vi "CreateShearRampStepVisualizationGraph.vi"(8 "Step Duration":dbl, 9 "Final Value":dbl, 10 "Initial Value":dbl, 11 "Number of Points":i32) -> (2 "Shear Step Array":dbl[][](array[numeric]), 3 "XY Graph":cluster{dbl[], "Ramp Pattern":dbl[]}(graph))   [LabVIEW 2021]
uses:
  <vilib>/Analysis/1siggen.llb/Ramp Pattern by Samples.vi
  <vilib>/Analysis/NI_AALBase.lvlib
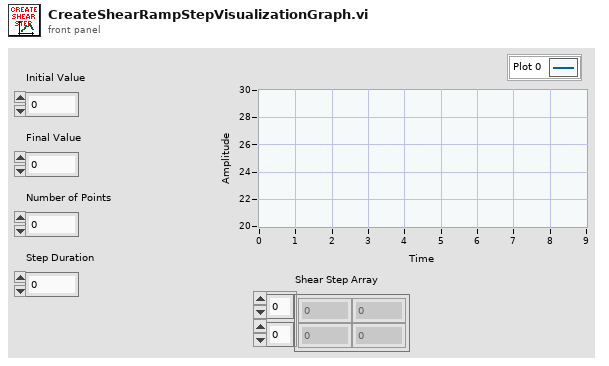
[diagram p1: front panel]
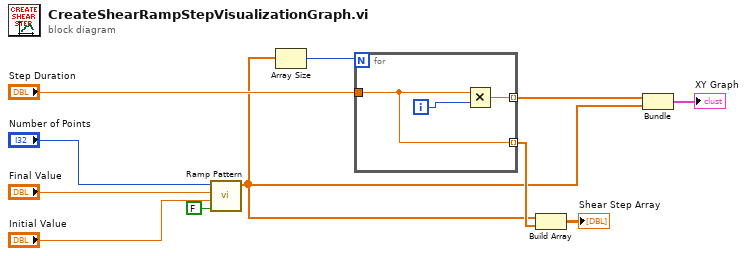
[diagram p0: block diagram]
diagram:
  n1 = call-poly <vilib>:"Ramp Pattern.vi"("exclude end?"=FALSE, "start"="Initial Value", "end"="Final Value", "samples"="Number of Points") -> ("Ramp Pattern"=w2:dbl[])  [unwired: 6 in, 1 out]
  n2 = Array Size(array=w2) -> (size(s)=w1:i32)
  n3 = for {
    N: w1 -> [_]
    tunnel: "Step Duration" -> [w13]
    tunnel: [w14] -> w11 mode=indexing
    tunnel: [w13] -> w4 mode=indexing
    i -> [w12]
    n4 = Multiply(x=w13, y=w12) -> (x*y=w14:dbl)
  }
  n5 = Build Array(w2, w4) -> (→"Shear Step Array":dbl[][])
  n6 = Bundle(w11, "Ramp Pattern"=w2) -> (→"XY Graph":cluster{dbl[], "Ramp Pattern":dbl[]})  [unwired: 1 in]
